vi "Config.Read Station Info.vi"(8 "error in (no error)":errorcluster, 11 "Local Station Config File":path) -> (0 "error out":errorcluster, 1 "Disable SN Route Ck":bool, 3 "Station":T1, 4 "Default Seq":string)   [LabVIEW 2018]
uses:
  Results/Result XML/TestResult.Station Info.ctl
  Results/Result XML/TestResult.HW Item.ctl
  Results/Result XML/TestResult.SW Item.ctl
  <vilib>/Utility/config.llb/Read Key (String).vi
  <vilib>/Utility/config.llb/Read Key (Boolean).vi
  <vilib>/Utility/config.llb/NI_LVConfig.lvlib
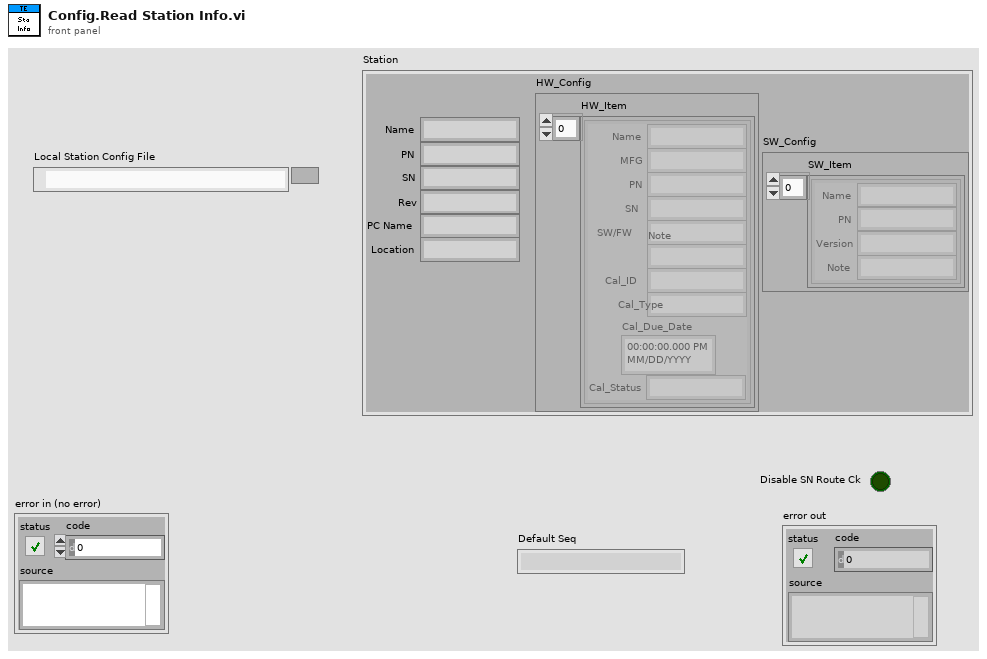
[diagram p1: front panel]
types:
  T1 = typedef "TestResult.Station Info.ctl" = cluster{"Name":string, "PN":string, "SN":string, "Rev":string, "PC Name":string, "Location":string, "HW_Config":cluster{"HW_Item":T2[]}, "SW_Config":cluster{"SW_Item":T3[]}}
  T2 = typedef "TestResult.HW Item.ctl" = cluster{"Name":string, "MFG":string, "PN":string, "SN":string, "SW/FW":string, "Note":string, "Cal_ID":string, "Cal_Type":string, "Cal_Due_Date":timestamp, "Cal_Status":string}
  T3 = typedef "TestResult.SW Item.ctl" = cluster{"Name":string, "PN":string, "Version":string, "Note":string}
  T4 = typedef "NI_LVConfig.lvlib/Config Data RefNum.ctl" = refnum<k1>
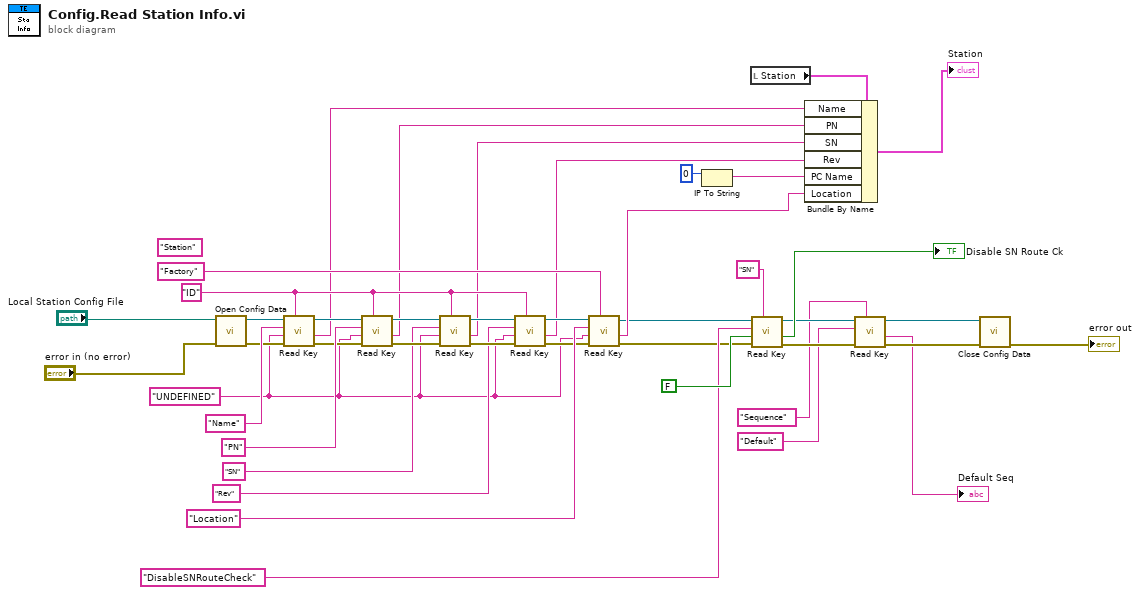
[diagram p0: block diagram]
diagram:
  w14 = "UNDEFINED"
  (unwired) "Station"
  w27 = "ID"
  n1 = call <vilib>:"Open Config Data.vi"("error in (no error)"="error in (no error)", "configuration file path"="Local Station Config File") -> ("error out"=w36:errorcluster, "refnum"=w39:T4)  [unwired: 7 in, 1 out]
  n2 = call-poly <vilib>:"Read Key.vi"("section"=w27, "error in (no error)"=w36, "default value"=w14, "key"="Name", "refnum"=w39) -> ("error out"=w37:errorcluster, "value"=w21:string, "refnum out"=w40:T4)  [unwired: 3 in, 1 out]
  n3 = call-poly <vilib>:"Read Key.vi"("section"=w27, "error in (no error)"=w37, "default value"=w14, "key"="PN", "refnum"=w40) -> ("error out"=w38:errorcluster, "value"=w18:string, "refnum out"=w41:T4)  [unwired: 3 in, 1 out]
  n4 = call-poly <vilib>:"Read Key.vi"("section"=w27, "error in (no error)"=w38, "default value"=w14, "key"="SN", "refnum"=w41) -> ("error out"=w31:errorcluster, "value"=w17:string, "refnum out"=w32:T4)  [unwired: 3 in, 1 out]
  n5 = call-poly <vilib>:"Read Key.vi"("section"=w27, "error in (no error)"=w31, "default value"=w14, "key"="Rev", "refnum"=w32) -> ("error out"=w30:errorcluster, "value"=w26:string, "refnum out"=w29:T4)  [unwired: 3 in, 1 out]
  n6 = call-poly <vilib>:"Read Key.vi"("section"="Factory", "error in (no error)"=w30, "default value"=w14, "key"="Location", "refnum"=w29) -> ("error out"=w1:errorcluster, "value"=w22:string, "refnum out"=w2:T4)  [unwired: 3 in, 1 out]
  n7 = IP To String(2:u32 0 ("net address")) -> (0:w15:string)  [unwired: 1 in]
  n8 = local read "Station"() -> (w24:T1)
  n9 = call-poly <vilib>:"Read Key.vi"("section"="SN", "error in (no error)"=w1, "default value"=FALSE, "key"="DisableSNRouteCheck", "refnum"=w2) -> ("error out"=w9:errorcluster, "value"=→"Disable SN Route Ck":bool, "refnum out"=w10:T4)  [unwired: 3 in, 1 out]
  n10 = Bundle By Name(cluster=w24, "Name"=w21, "PN"=w18, "SN"=w17, "Rev"=w26, "PC Name"=w15, "Location"=w22) -> (→"Station":T1)
  n11 = call-poly <vilib>:"Read Key.vi"("section"="Sequence", "error in (no error)"=w9, "key"="Default", "refnum"=w10) -> ("error out"=w8:errorcluster, "value"=→"Default Seq":string, "refnum out"=w7:T4)  [unwired: 4 in, 1 out]
  n12 = call <vilib>:"Close Config Data.vi"("error in (no error)"=w8, "refnum"=w7) -> ("error out"=→"error out":errorcluster)  [unwired: 8 in, 1 out]
